vi "postionSet.vi"(3 "error in (no error)":errorcluster, 4 "Pos in":dbl[](array[numeric]), 5 "UART PORT in":refnum<visa-resource-name>) -> (0 "error out":errorcluster, 1 "Pos out":dbl[](array[numeric]), 2 "UART PORT out":refnum<visa-resource-name>)   [LabVIEW 2016]
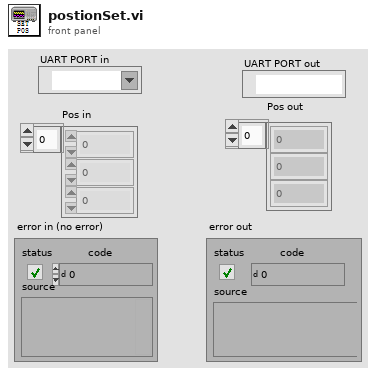
[diagram p1: front panel]
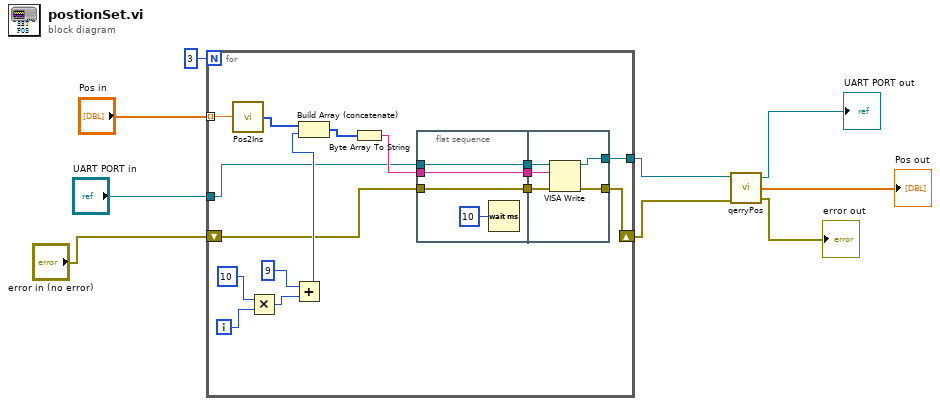
[diagram p0: block diagram]
diagram:
  n1 = for {
    N: 3 -> [_]
    tunnel: "Pos in" -> [w25] mode=indexing
    tunnel: "UART PORT in" -> [w16]
    shift-right: [w11] -> w5
    shift-left: "error in (no error)" -> [w15]
    tunnel: [w10] -> w4
    i -> [w24]
    n2 = call "Pos2Ins.vi"("Pos"=w25) -> ("Ins"=w20:i32[])
    n3 = Multiply(x=10, y=w24) -> (x*y=w22:i32)
    n4 = Add(x=9, y=w22) -> (x+y=w19:i32)
    n5 = Build Array (concatenate)(w20, w19) -> (w18:i32[])
    n6 = Byte Array To String(unsigned byte array=w18) -> (string=w17:string)
    n7 = flat-sequence {
      tunnel: w15 -> [w27]
      tunnel: w16 -> [w28]
      tunnel: w17 -> [w29]
      tunnel: [w29] -> w14
      tunnel: [w28] -> w13
      tunnel: [w27] -> w12
      tunnel: w14 -> [w34]
      tunnel: w13 -> [w33]
      tunnel: w12 -> [w32]
      tunnel: [w31] -> w11
      tunnel: [w30] -> w10
      frame #0 {
        n8 = Wait (ms)(milliseconds to wait=u32 10) -> ()  [unwired: 1 out]
      }
      frame #1 {
        n9 = VISA Write(VISA resource name=w33, write buffer=w34, error in (no error)=w32) -> (VISA resource name out=w30:refnum<visa-resource-name>, error out=w31:errorcluster)  [unwired: 1 out]
      }
    }
  }
  n10 = call "qerryPos.vi"("error in (no error)"=w5, "UART in"=w4) -> ("error out"=→"error out":errorcluster, "Array"=→"Pos out":dbl[], "UART out"=→"UART PORT out":refnum<visa-resource-name>)  [unwired: 2 in]
